vi "PlotGraphs.vi"(0 "Game in":refnum<class "Game.lvclass">, 5 "id 1":dbl, 7 "id 2":dbl, 9 "id 3":dbl, 11 "error in (no error)":errorcluster) -> (3 "ball":dbl(graph), 4 "Game out":refnum<class "Game.lvclass">, 6 "Robot 1":T1(graph), 8 "Robot 2":T1(graph), 10 "Robot 3":T1(graph), 15 "error out":errorcluster)   [LabVIEW 2018, in "Game.lvclass"]
uses:
  Game.lvclass
  Robot_class/Robot.lvclass
  Game.lvclass/Game.ctl
  Team_class/Team.lvclass/Team.ctl
  Ball_class/Ball.lvclass/Ball.ctl
  Robot_class/Robot.lvclass/Robot.ctl
  Robot_class/Read v_norm.vi
  Robot_class/Read v_tang.vi
  Robot_class/Read vx_desired.vi
  Robot_class/Read vy_desired.vi
  Read Utilities.lvclass.vi
  Read KeeperTeam.vi
  Read OffensiveTeam.vi
  Read DefensiveTeam.vi
  Read BallRef.vi
  Ball_class/Read v_x.vi
  Ball_class/Read v_y.vi
  Team_class/Read RobotRef.vi
  Ally_class/Ally.lvclass
  C:/Users/Guilherme Moreira/OneDrive/Dokumente/SSL_AI_nicolas/SSL_AI/Team_class/Team.lvclass
  Utilities_class/Utilities.lvclass
  Ball_class/Ball.lvclass
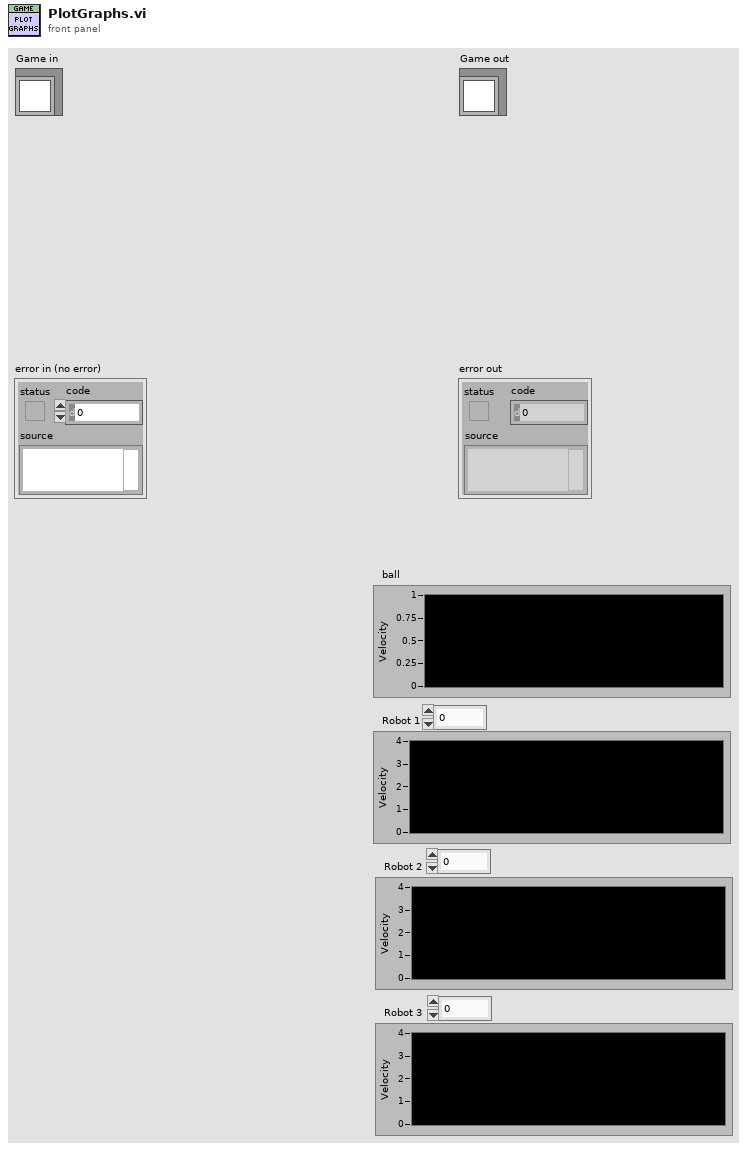
[diagram p1: front panel]
types:
  T1 = cluster{"Modulo":dbl, "Modulo":dbl, "Modulo":dbl}
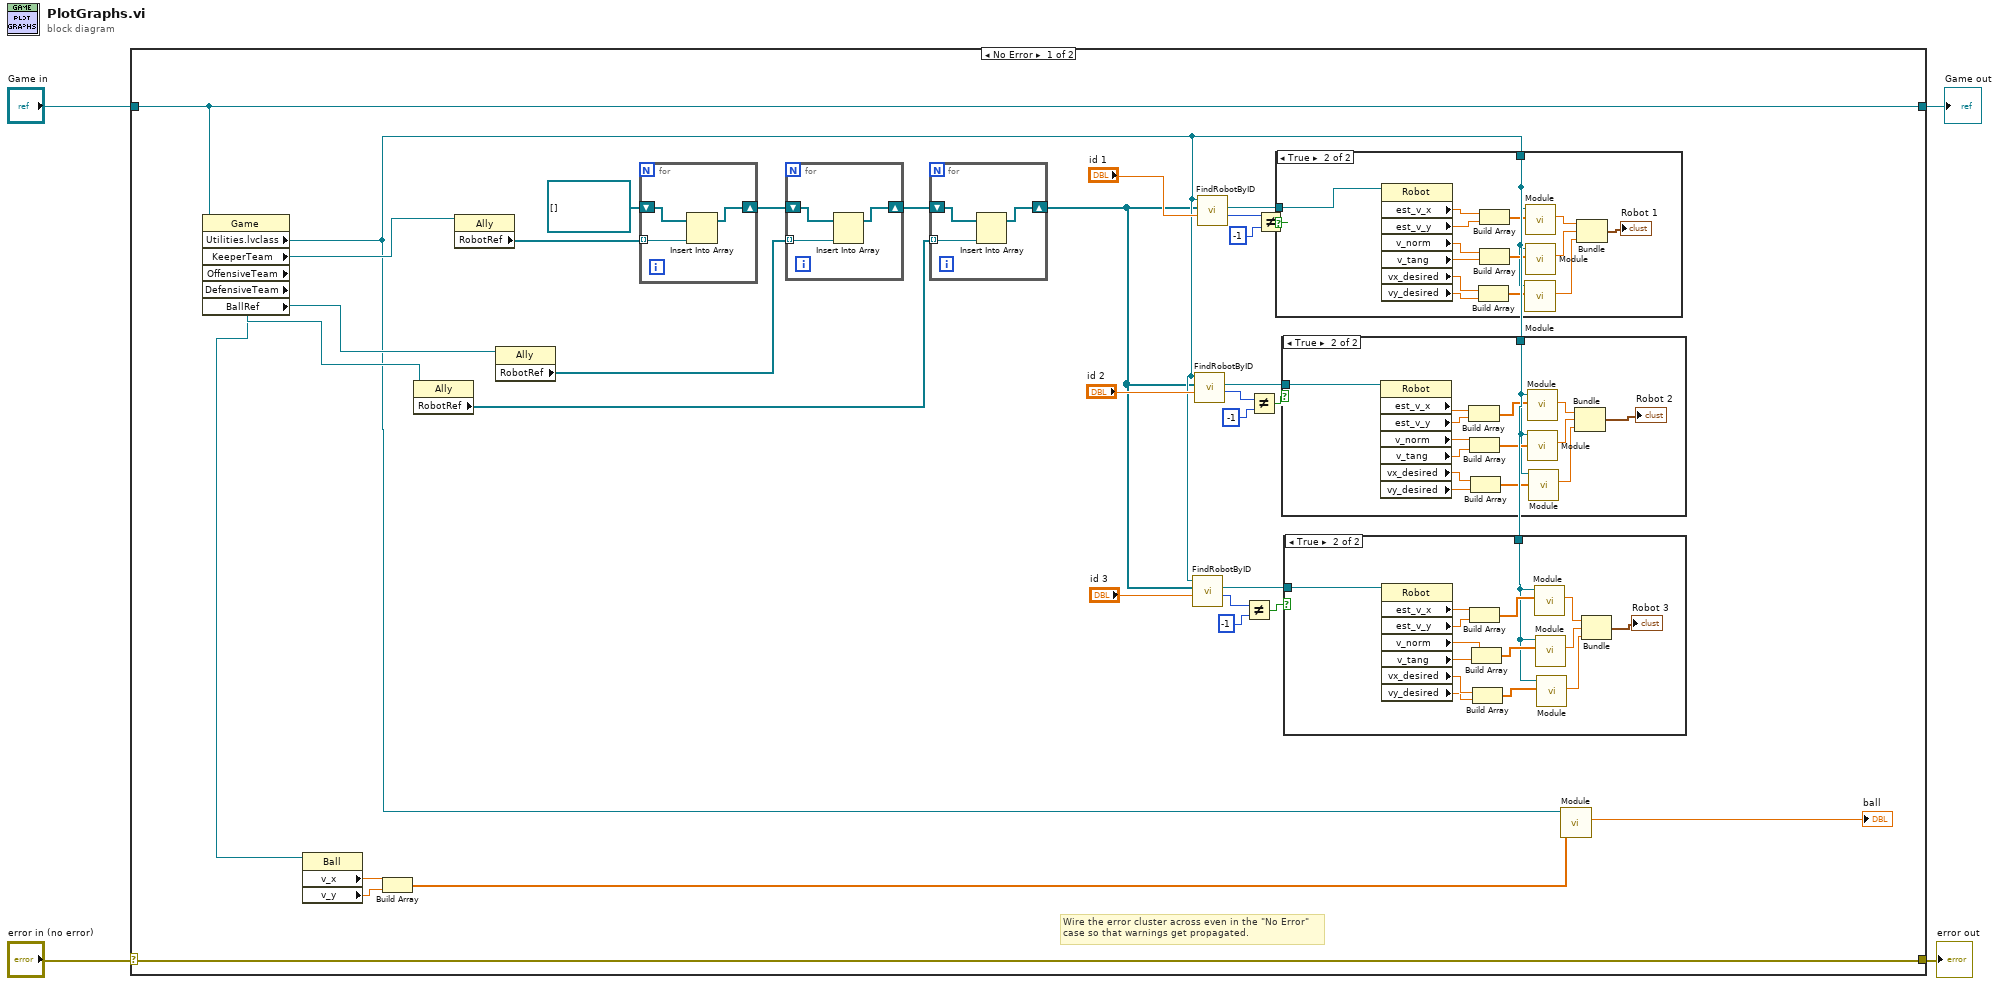
[diagram p0: block diagram]
diagram:
  n1 = case shown="No Error" "error in (no error)" {
    selector: "error in (no error)" -> [w37 w93]
    tunnel: [w37 w93] -> w3
    tunnel: [w28 w92] -> w1
    tunnel: "Game in" -> [w28 w92]
    frame No Error {
      # "Wire the error cluster across even in the \"No Error\"\ncase so that warnings get propagated."
      n2 = property class="Game"(reference=w28) -> ("Utilities.lvclass"=w15:refnum<class "Utilities.lvclass">, "KeeperTeam"=w36:refnum<class "Ally.lvclass">, "OffensiveTeam"=w35:refnum<class "Ally.lvclass">, "DefensiveTeam"=w34:refnum<class "Ally.lvclass">, "BallRef"=w33:refnum<class "Ball.lvclass">)  [unwired: 1 in, 2 out]
      n3 = property class="Ball"(reference=w33) -> ("v_x"=w32:dbl, "v_y"=w31:dbl)  [unwired: 1 in, 2 out]
      n4 = Build Array(w32, w31) -> (w30:dbl[])
      n5 = property class="Ally"(reference=w34) -> ("RobotRef"=w22:refnum<class "Robot.lvclass">[])  [unwired: 1 in, 2 out]
      n6 = property class="Ally"(reference=w36) -> ("RobotRef"=w27:refnum<class "Robot.lvclass">[])  [unwired: 1 in, 2 out]
      n7 = property class="Ally"(reference=w35) -> ("RobotRef"=w24:refnum<class "Robot.lvclass">[])  [unwired: 1 in, 2 out]
      n8 = for {
        tunnel: w27 -> [w46] mode=indexing
        shift-right: [w44] -> w25
        shift-left: refnum<class "Robot.lvclass">[] [] -> [w45]
        n9 = Insert Into Array(array=w45, new element=w46) -> (w44:refnum<class "Robot.lvclass">[])  [unwired: 1 in]
      }
      n10 = for {
        tunnel: w24 -> [w43] mode=indexing
        shift-right: [w41] -> w23
        shift-left: w25 -> [w42]
        n11 = Insert Into Array(array=w42, new element=w43) -> (w41:refnum<class "Robot.lvclass">[])  [unwired: 1 in]
      }
      n12 = for {
        tunnel: w22 -> [w40] mode=indexing
        shift-right: [w38] -> w5
        shift-left: w23 -> [w39]
        n13 = Insert Into Array(array=w39, new element=w40) -> (w38:refnum<class "Robot.lvclass">[])  [unwired: 1 in]
      }
      n14 = call-dynamic "FindRobotByID.vi"("id"="id 3", "RobotRef"=w5, "Utilities in"=w15) -> ("index"=w9:i32, "Robot"=w16:refnum<class "Robot.lvclass">)  [unwired: 5 in, 2 out]
      n15 = call-dynamic "FindRobotByID.vi"("id"="id 2", "RobotRef"=w5, "Utilities in"=w15) -> ("index"=w10:i32, "Robot"=w18:refnum<class "Robot.lvclass">)  [unwired: 5 in, 2 out]
      n16 = call-dynamic "FindRobotByID.vi"("id"="id 1", "RobotRef"=w5, "Utilities in"=w15) -> ("index"=w14:i32, "Robot"=w20:refnum<class "Robot.lvclass">)  [unwired: 5 in, 2 out]
      n17 = Not Equal?(x=w9, y=-1) -> (x != y?=w8:bool)
      n18 = Not Equal?(x=w10, y=-1) -> (x != y?=w7:bool)
      n19 = Not Equal?(x=w14, y=-1) -> (x != y?=w6:bool)
      n20 = case shown="True" w6 {
        tunnel: w20 -> [_ w91]
        tunnel: w15 -> [_ w81]
        frame False {
        }
        frame True {
          n21 = property class="Robot"(reference=w91) -> ("est_v_x"=w90:dbl, "est_v_y"=w89:dbl, "v_norm"=w86:dbl, "v_tang"=w85:dbl, "vx_desired"=w78:dbl, "vy_desired"=w77:dbl)  [unwired: 1 in, 2 out]
          n22 = Build Array(w78, w77) -> (w79:dbl[])
          n23 = Build Array(w90, w89) -> (w88:dbl[])
          n24 = Build Array(w86, w85) -> (w87:dbl[])
          n25 = call-dynamic "Module.vi"("2D vector"=w79, "Utilities in"=w81) -> ("Modulo"=w80:dbl)  [unwired: 7 in, 2 out]
          n26 = call-dynamic "Module.vi"("2D vector"=w88, "Utilities in"=w81) -> ("Modulo"=w83:dbl)  [unwired: 7 in, 2 out]
          n27 = call-dynamic "Module.vi"("2D vector"=w87, "Utilities in"=w81) -> ("Modulo"=w84:dbl)  [unwired: 7 in, 2 out]
          n28 = Bundle("Modulo"=w83, "Modulo"=w84, "Modulo"=w80) -> (→"Robot 1":T1)  [unwired: 1 in]
        }
      }
      n29 = case shown="True" w7 {
        tunnel: w18 -> [_ w76]
        tunnel: w15 -> [_ w64]
        frame False {
        }
        frame True {
          n30 = property class="Robot"(reference=w76) -> ("est_v_x"=w74:dbl, "est_v_y"=w75:dbl, "v_norm"=w72:dbl, "v_tang"=w71:dbl, "vx_desired"=w63:dbl, "vy_desired"=w62:dbl)  [unwired: 1 in, 2 out]
          n31 = Build Array(w74, w75) -> (w73:dbl[])
          n32 = Build Array(w72, w71) -> (w70:dbl[])
          n33 = Build Array(w63, w62) -> (w66:dbl[])
          n34 = call-dynamic "Module.vi"("2D vector"=w73, "Utilities in"=w64) -> ("Modulo"=w69:dbl)  [unwired: 7 in, 2 out]
          n35 = call-dynamic "Module.vi"("2D vector"=w70, "Utilities in"=w64) -> ("Modulo"=w68:dbl)  [unwired: 7 in, 2 out]
          n36 = call-dynamic "Module.vi"("2D vector"=w66, "Utilities in"=w64) -> ("Modulo"=w65:dbl)  [unwired: 7 in, 2 out]
          n37 = Bundle("Modulo"=w69, "Modulo"=w68, "Modulo"=w65) -> (→"Robot 2":T1)  [unwired: 1 in]
        }
      }
      n38 = case shown="True" w8 {
        tunnel: w16 -> [_ w61]
        tunnel: w15 -> [_ w50]
        frame False {
        }
        frame True {
          n39 = property class="Robot"(reference=w61) -> ("est_v_x"=w60:dbl, "est_v_y"=w59:dbl, "v_norm"=w57:dbl, "v_tang"=w56:dbl, "vx_desired"=w49:dbl, "vy_desired"=w48:dbl)  [unwired: 1 in, 2 out]
          n40 = Build Array(w60, w59) -> (w58:dbl[])
          n41 = Build Array(w57, w56) -> (w55:dbl[])
          n42 = Build Array(w49, w48) -> (w51:dbl[])
          n43 = call-dynamic "Module.vi"("2D vector"=w58, "Utilities in"=w50) -> ("Modulo"=w53:dbl)  [unwired: 7 in, 2 out]
          n44 = call-dynamic "Module.vi"("2D vector"=w55, "Utilities in"=w50) -> ("Modulo"=w54:dbl)  [unwired: 7 in, 2 out]
          n45 = call-dynamic "Module.vi"("2D vector"=w51, "Utilities in"=w50) -> ("Modulo"=w47:dbl)  [unwired: 7 in, 2 out]
          n46 = Bundle("Modulo"=w53, "Modulo"=w54, "Modulo"=w47) -> (→"Robot 3":T1)  [unwired: 1 in]
        }
      }
      n47 = call-dynamic "Module.vi"("2D vector"=w30, "Utilities in"=w15) -> ("Modulo"=→"ball":dbl)  [unwired: 7 in, 2 out]
    }
    frame Error {
    }
  }
  "error out" <- w3
  "Game out" <- w1
